vi "Emballage_BDD_date.vi"(11 "Date":string) -> (1 "Date_jour":string, 2 "Date_mois":string, 3 "Date_annee":string)   [LabVIEW 2020]
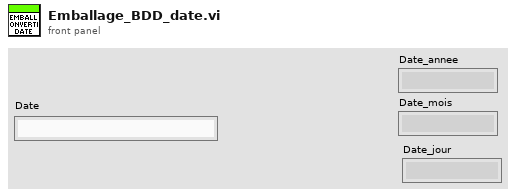
[diagram p1: front panel]
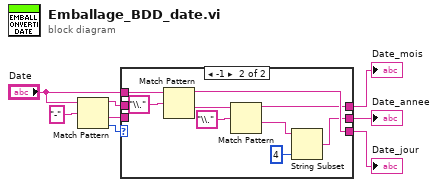
[diagram p0: block diagram]
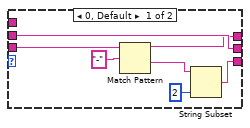
[diagram p2: hidden frame]
diagram:
  n1 = Match Pattern(string="Date", regular expression="-") -> (before substring=w4:string, after substring=w3:string, offset past match=w7:i32)  [unwired: 1 in, 1 out]
  n2 = case shown="-1" w7 {
    tunnel: "Date" -> [_ w23]
    tunnel: [w15 w17] -> w5
    tunnel: w4 -> [w15 _]
    tunnel: w3 -> [w13 _]
    tunnel: [w12 w19] -> w2
    tunnel: [w9 w22] -> w1
    frame 0, Default {
      n3 = Match Pattern(string=w13, regular expression="-") -> (before substring=w12:string, after substring=w10:string)  [unwired: 1 in, 2 out]
      n4 = String Subset(string=w10, length (rest)=2 ("length (rest)")) -> (substring=w9:string)  [unwired: 1 in]
    }
    frame -1 {
      n5 = Match Pattern(string=w23, regular expression="\\.") -> (before substring=w22:string, after substring=w20:string)  [unwired: 1 in, 2 out]
      n6 = Match Pattern(string=w20, regular expression="\\.") -> (before substring=w19:string, after substring=w18:string)  [unwired: 1 in, 2 out]
      n7 = String Subset(string=w18, length (rest)=4 ("length (rest)")) -> (substring=w17:string)  [unwired: 1 in]
    }
  }
  "Date_annee" <- w5
  "Date_mois" <- w2
  "Date_jour" <- w1
